vi "Trigger Delay Test.vi"() -> ()   [LabVIEW 2016]
uses:
  <instrlib>/niScope/Controls/niScope trigger source digital.ctl
  <instrlib>/niScope/Configure/Trigger/niScope Configure Trigger Digital.vi
  <instrlib>/niScope/Acquire/Fetch/niScope Multi Fetch Binary 16.vi
  <instrlib>/niScope/Acquire/Fetch/niScope Multi Fetch WDT.vi
panel:
  in  "Fetch:Fetch Relative To 2":i32(ring)=482 items=["Start"=482, "Trigger"=483, "Pretrigger"=477, "Now"=481, "Read Pointer"=388]
  in  "Watch backlog":bool
  in  "Read I16?":bool
  out "Fetch:Fetch Relative To":i32(ring)=482 items=["Start"=482, "Trigger"=483, "Pretrigger"=477, "Now"=481, "Read Pointer"=388]
  out "Fetch:Fetch Offset":i32
  out "Finished":bool
  in  "vertical range":dbl=10.0 format="%.2f"
  in  "trigger source":T1="VAL_RTSI_0"
  in  "min record length":i32=100000
  in  "reference position":dbl=50.0 format="%.1f"
  in  "min sample rate":dbl=1000000.0 format="%^.2e"
  in  "channels":string="0"
  in  "resource name":refnum<k15>="5105-PCI"
  out "Waveform Graph":waveform(dbl)[](graph)
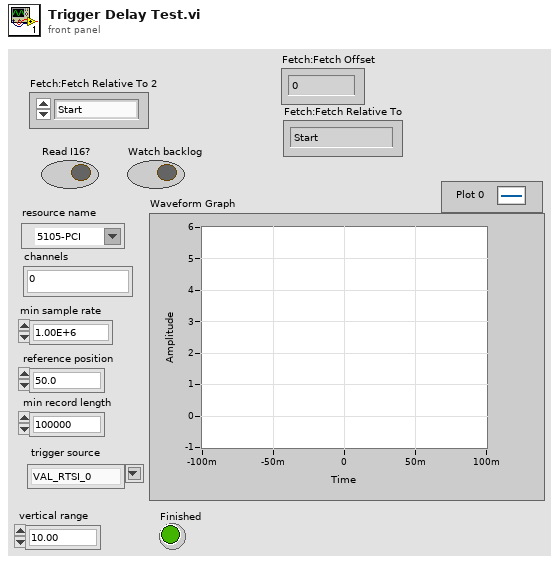
[diagram p1: front panel]
types:
  T1 = typedef "niScope trigger source digital.ctl" = string
  T2 = cluster{"actualSamples":i32, "absoluteInitialX":dbl, "relativeInitialX":dbl, "xIncrement":dbl, "offset":dbl, "gain":dbl, "reserved1":dbl, "reserved2":dbl}[]
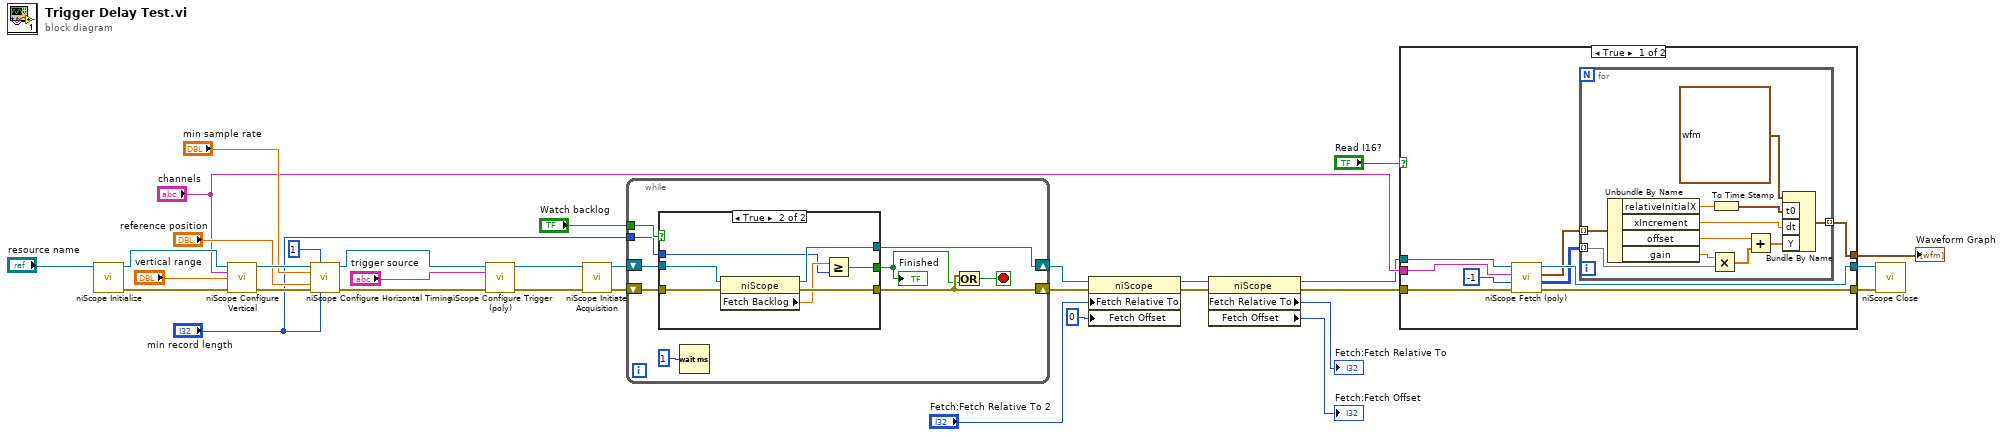
[diagram p0: block diagram]
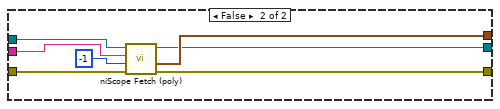
[diagram p2: hidden frame]
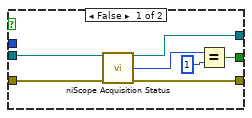
[diagram p3: hidden frame]
diagram:
  n1 = call <instrlib>:"niScope Initialize.vi"("resource name"="resource name") -> ("instrument handle"=w32:refnum<k15>, "error out"=w31:errorcluster)  [unwired: 13 in]
  n2 = call <instrlib>:"niScope Configure Vertical.vi"("instrument handle"=w32, "channels"="channels", "vertical range"="vertical range", "error in"=w31) -> ("instrument handle out"=w30:refnum<k15>, "error out"=w29:errorcluster)  [unwired: 10 in]
  n3 = call <instrlib>:"niScope Configure Horizontal Timing.vi"("instrument handle"=w30, "number of records"=1, "min sample rate"="min sample rate", "reference position"="reference position", "error in"=w29, "min record length"="min record length") -> ("instrument handle out"=w26:refnum<k15>, "error out"=w25:errorcluster)  [unwired: 8 in]
  n4 = call-poly <instrlib>:"niScope Configure Trigger (poly).vi"("instrument handle"=w26, "trigger source"="trigger source", "error in"=w25) -> ("instrument handle out"=w21:refnum<k15>, "error out"=w20:errorcluster)  [unwired: 11 in]
  n5 = call <instrlib>:"niScope Initiate Acquisition.vi"("instrument handle"=w21, "error in"=w20) -> ("instrument handle out"=w19:refnum<k15>, "error out"=w18:errorcluster)  [unwired: 12 in]
  n6 = while {
    shift-right: [w39] -> w17
    shift-left: w18 -> [w41]
    shift-right: [w40] -> w6
    shift-left: w19 -> [w42]
    tunnel: "Watch backlog" -> [w35]
    tunnel: "min record length" -> [w34]
    stop <- w37 stop-if-true
    n7 = case shown="True" w35 {
      tunnel: w42 -> [w49 w55]
      tunnel: w41 -> [w48 w54]
      tunnel: [w47 w53] -> w40
      tunnel: [w44 w56] -> w39
      tunnel: [w43 w52] -> w38
      tunnel: w34 -> [_ w50]
      frame False {
        n8 = call <instrlib>:"niScope Acquisition Status.vi"("instrument handle"=w49, "error in"=w48) -> ("instrument handle out"=w47:refnum<k15>, "acquisition status"=w45:i32, "error out"=w44:errorcluster)  [unwired: 11 out]
        n9 = Equal?(x=w45, y=1) -> (x = y?=w43:bool)
      }
      frame True {
        n10 = property class="niScope"(reference=w55, error in=w54) -> (reference out=w53:refnum<k15>, error out=w56:errorcluster, "Fetch Backlog"=w51:dbl)
        n11 = Greater Or Equal?(x=w51, y=w50) -> (x >= y?=w52:bool)
      }
    }
    "Finished" <- w38
    n12 = Wait (ms)(milliseconds to wait=u32 1) -> ()  [unwired: 1 out]
    n13 = Or(x=w39, y=w38) -> (x .or. y?=w37:bool)
  }
  n14 = property class="niScope"(reference=w6, error in=w17, "Fetch Relative To"="Fetch:Fetch Relative To 2", "Fetch Offset"=0 ("Fetch:Fetch Offset")) -> (reference out=w5:refnum<k15>, error out=w7:errorcluster)
  n15 = property class="niScope"(reference=w5, error in=w7) -> (reference out=w11:refnum<k15>, error out=w12:errorcluster, "Fetch Relative To"=→"Fetch:Fetch Relative To":i32, "Fetch Offset"=→"Fetch:Fetch Offset":i32)
  n16 = case shown="True" "Read I16?" {
    tunnel: [w60 w83] -> w16
    tunnel: [w65 w82] -> w15
    tunnel: [w64 w81] -> w14
    tunnel: "channels" -> [w63 w80]
    tunnel: w12 -> [w62 w79]
    tunnel: w11 -> [w61 w78]
    frame True {
      n17 = call-poly <instrlib>:"niScope Fetch (poly).vi"("error in"=w62, "numSamples"=-1, "channels"=w63, "instrument handle"=w61) -> ("error out"=w64:errorcluster, "wfm"=w59:i16[][], "wfm info"=w57:T2, "instrument handle out"=w65:refnum<k15>)  [unwired: 4 in]
      n18 = for {
        tunnel: [w72] -> w60 mode=indexing
        tunnel: w59 -> [w70] mode=indexing
        tunnel: w57 -> [w66] mode=indexing
        n19 = Unbundle By Name(w66) -> ("relativeInitialX"=w75:dbl, "xIncrement"=w73:dbl, "offset"=w68:dbl, "gain"=w71:dbl)
        n20 = Multiply(x=w71, y=w70) -> (x*y=w69:dbl[])
        n21 = To Time Stamp(1:w75) -> (0:w74:timestamp)
        n22 = Add(x=w68, y=w69) -> (x+y=w67:dbl[])
        n23 = Bundle By Name(cluster=waveform(dbl) {"t0"=timestamp(0 s since 1904-01-01), "dt"=0.0, "Y"=[]} ("wfm"), "t0"=w74, "dt"=w73, "Y"=w67) -> (w72:waveform(dbl))
      }
    }
    frame False {
      n24 = call-poly <instrlib>:"niScope Fetch (poly).vi"("error in"=w79, "numSamples"=-1, "channels"=w80, "instrument handle"=w78) -> ("error out"=w81:errorcluster, "wfm"=w83:waveform(dbl)[], "instrument handle out"=w82:refnum<k15>)  [unwired: 4 in, 1 out]
    }
  }
  "Waveform Graph" <- w16
  n25 = call <instrlib>:"niScope Close.vi"("instrument handle"=w15, "error in"=w14) -> ()  [unwired: 14 out]
